vi "ROI entry-ROI text overlay.vi"(6 "ROI properties":T1 {"ROI group ID" format="%#_6f"; "Laser Power (%)" format="%#_6f"; "Zoom" format="%#_6f"; "Frame Size" format="%#_6f"; "Number of lines" format="%#_6f"; "Composite ID" format="%#_6f"; "Angle (deg)" format="%#_6f"; "ROI Time (ns)" format="%#_6f"; "ROI ID" format="%#_6f"; "Pixels in ROI" format="%#_6f"; "ROI index" format="%#_6f"; "Z stop" format="%#_6f"; "Y stop" format="%#_6f"; "X stop" format="%#_6f"; "Z start" format="%#_6f"; "X start" format="%#_6f"; "Y start" format="%#_6f"}, 8 "Error in (no error)":errorcluster, 9 "Point":cluster{"X":i32, "Y":i32}, 10 "Rect. text colour":u32, 11 "Refnum in":T2) -> (0 "error out":errorcluster, 3 "Refnum out":T2)   [LabVIEW 2013]
uses:
  <vilib>/vision/Image Controls.llb/IMAQ Image.ctl
  Visualisation/Functional Imaging Viewer/Typedefs/ROI parameters data type.ctl
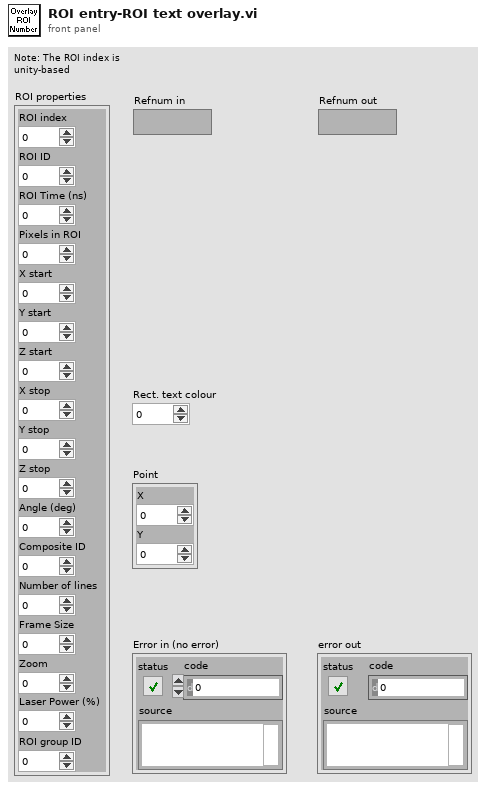
[diagram p1: front panel]
types:
  T1 = typedef "ROI parameters data type.ctl" = cluster{"ROI index":dbl, "ROI ID":dbl, "ROI Time (ns)":dbl, "Pixels in ROI":dbl, "X start":dbl, "Y start":dbl, "Z start":dbl, "X stop":dbl, "Y stop":dbl, "Z stop":dbl, "Angle (deg)":dbl, "Composite ID":dbl, "Number of lines":dbl, "Frame Size":dbl, "Zoom":dbl, "Laser Power (%)":dbl, "ROI group ID":dbl}
  T2 = typedef "IMAQ Image.ctl" = refnum<image>
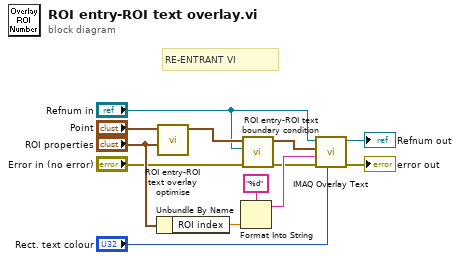
[diagram p0: block diagram]
diagram:
  # "RE-ENTRANT VI"
  n1 = Unbundle By Name("ROI properties") -> ("ROI index"=w8:dbl)
  n2 = call "ROI entry-ROI text overlay optimise.vi"("ROI properties"="ROI properties", "XY coordinates"="Point") -> ("XY coordinates"=w5:cluster{"X":i32, "Y":i32})  [unwired: 9 in]
  n3 = Format Into String(format string="%d", w8) -> (resulting string=w7:string)  [unwired: 2 in, 1 out]
  n4 = call "ROI entry-ROI text boundary condition.vi"("Error in (no error)"="Error in (no error)", "Image"="Refnum in", "XY coordinates in"=w5) -> ("error out"=w2:errorcluster, "XY coordinates out"=w4:cluster{"X":i32, "Y":i32})  [unwired: 7 in]
  n5 = call "IMAQ Overlay Text"("Text Color (black)"="Rect. text colour", "error in (no error)"=w2, "String"=w7, "Origin"=w4, "Image"="Refnum in") -> ("error out"=→"error out":errorcluster, "Image Out"=→"Refnum out":T2)  [unwired: 5 in]
